vi "RDV-linkPlotVisibility.vi"(8 "error in (no error)":errorcluster, 11 "RDV-Reflection_Data_viewer in":refnum<class "RDV-Reflection_Data_viewer.lvclass">) -> (0 "error out":errorcluster, 3 "RDV-Reflection_Data_viewer out":refnum<class "RDV-Reflection_Data_viewer.lvclass">)   [LabVIEW 2020, in "RDV-Reflection_Data_viewer.lvclass"]
uses:
  RDV-Reflection_Data_viewer.lvclass
  RDV-Reflection_Data_viewer.lvclass/RDV-Reflection_Data_viewer.ctl
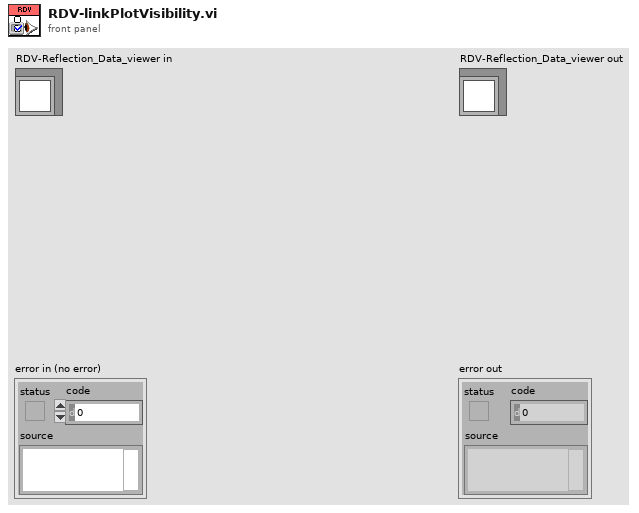
[diagram p1: front panel]
types:
  T1 = typedef "RDV-Reflection_Data_viewer.lvclass/RDV-XY_GRAPH_REFS.ctl" = cluster{"Reflection Real":refnum<vi>, "Reflection Imag":refnum<vi>, "Permittivity Real":refnum<vi>, "Permittivity Imag":refnum<vi>}
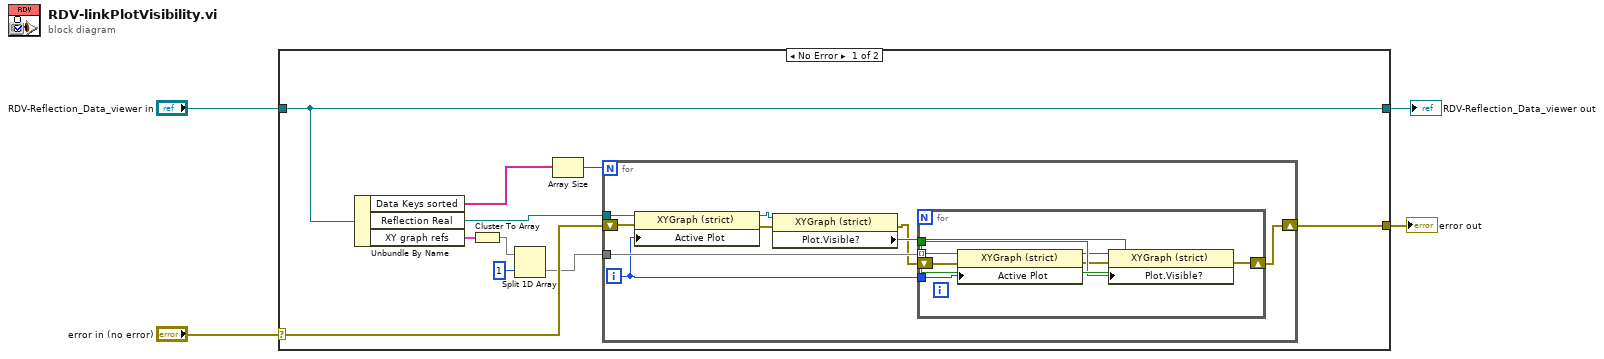
[diagram p0: block diagram]
diagram:
  n1 = case shown="No Error" "error in (no error)" {
    selector: "error in (no error)" -> [w10 w32]
    tunnel: [w11 w32] -> w3
    tunnel: [w14 w31] -> w1
    tunnel: "RDV-Reflection_Data_viewer in" -> [w14 w31]
    frame No Error {
      n2 = Unbundle By Name(w14) -> ("Data Keys sorted"=w13:string[], "Reflection Real"=w9:refnum<vi>, "XY graph refs"=w7:T1)
      n3 = Cluster To Array(cluster=w7) -> (array=w6:refnum<vi>[])
      n4 = Split 1D Array(array=w6, index=1) -> (second subarray=w5:refnum<vi>[])  [unwired: 1 out]
      n5 = Array Size(array=w13) -> (size(s)=w12:i32)
      n6 = for {
        N: w12 -> [_]
        tunnel: w5 -> [w23]
        tunnel: w9 -> [w21]
        shift-right: [w16] -> w11
        shift-left: w10 -> [w15]
        i -> [w19]
        n7 = property on="Property Node" class="XYGraph (strict)"(reference=w21, error in=w15, "Active Plot"=w19) -> (reference out=w20:refnum<vi>, error out=w17:errorcluster)
        n8 = property on="Property Node" class="XYGraph (strict)"(reference=w20, error in=w17) -> (error out=w18:errorcluster, "Plot.Visible?"=w22:bool)  [unwired: 1 out]
        n9 = for {
          tunnel: w22 -> [w30]
          tunnel: w23 -> [w29] mode=indexing
          tunnel: w19 -> [w26]
          shift-right: [w25] -> w16
          shift-left: w18 -> [w24]
          n10 = property on="Property Node" class="XYGraph (strict)"(reference=w29, error in=w24, "Active Plot"=w26) -> (reference out=w28:refnum<vi>, error out=w27:errorcluster)
          n11 = property on="Property Node" class="XYGraph (strict)"(reference=w28, error in=w27, "Plot.Visible?"=w30) -> (error out=w25:errorcluster)  [unwired: 1 out]
        }
      }
    }
    frame Error {
    }
  }
  "error out" <- w3
  "RDV-Reflection_Data_viewer out" <- w1
